vi "Get Variable Container.vi"(8 "error in (no error)":errorcluster, 10 "Type":T2, 11 "TSEngine in":refnum<class "Engine.lvclass">) -> (0 "error out":errorcluster, 2 "VariableContainer":T1, 3 "TSEngine out":refnum<class "Engine.lvclass">)   [LabVIEW 2019, in "HTS.lvlib" / "Engine.lvclass"]
uses:
  Engine.lvclass
  VariableContainer/VariableContainer.lvclass
  VariableContainer/Typedefs/Session Handle.ctl
  Variable Container Type.ctl
  Create VC Event Data.ctl
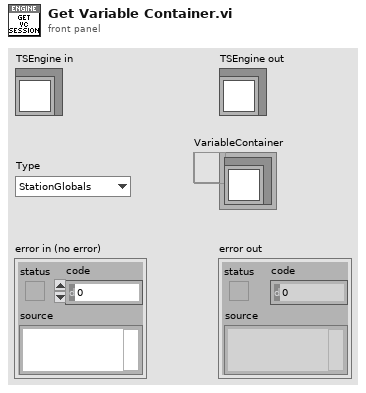
[diagram p1: front panel]
types:
  T1 = typedef "HTS.lvlib/VariableContainer.lvclass/Session Handle.ctl" = refnum<data-value>
  T2 = typedef "HTS.lvlib/Engine.lvclass/Variable Container Type.ctl" = enum16{"StationGlobals", "TemporaryGlobals", "NewPropertyObject"}
  T3 = typedef "HTS.lvlib/Engine.lvclass/Create VC Event Data.ctl" = cluster{"Type":T2, "Notifier":refnum<notifier>}
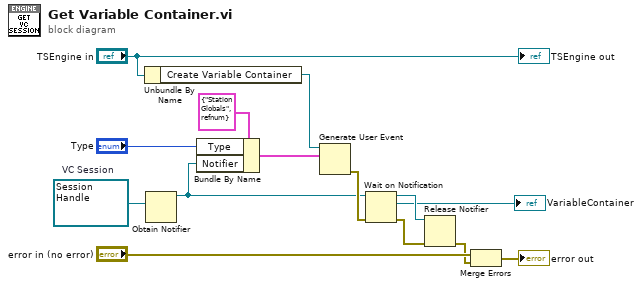
[diagram p0: block diagram]
diagram:
  w13 = T1 refnum  # VC Session
  n1 = Unbundle By Name("TSEngine in") -> ("Create Variable Container"=w9:refnum<user-event>)
  n2 = Obtain Notifier(notification data type=w13) -> (notifier out=w10:refnum<notifier>)  [unwired: 3 in, 2 out]
  n3 = Bundle By Name(cluster=T3 {"Type"=enum."StationGlobals", "Notifier"=refnum} ("Create Session Event Data"), "Type"="Type", "Notifier"=w10) -> (w8:T3)
  n4 = Generate User Event(user event=w9, event data cluster=w8) -> (error out=w14:errorcluster)  [unwired: 2 in, 1 out]
  n5 = Wait on Notification(notifier=w10, error in (no error)=w14) -> (notifier out=w5:refnum<notifier>, notification=→"VariableContainer":T1, error out=w4:errorcluster)  [unwired: 2 in, 1 out]
  n6 = Release Notifier(notifier=w5, error in (no error)=w4) -> (error out=w2:errorcluster)  [unwired: 1 in, 2 out]
  n7 = Merge Errors("error in (no error)", w2) -> (→"error out":errorcluster)
  "TSEngine out" <- "TSEngine in"
